vi "Insert Into Array (Boolean[]).vi"(9 "index":i32, 10 "Array":bool[](array[boolean]), 11 "JSON Value in":refnum<class "JSON Value.lvclass">) -> (3 "JSON Value out":refnum<class "JSON Value.lvclass">)   [LabVIEW 2017, in "JSON Value.lvclass"]
doc: "Inserts an element or subarray into a JSON array at the point you specify in index."
uses:
  JSON Value.lvclass
  Insert Into Array (Value[]).vi
  New JSON Value/New JSON (Boolean).vi
panel:
  out "error out":errorcluster
  in  "error in (no error)":errorcluster
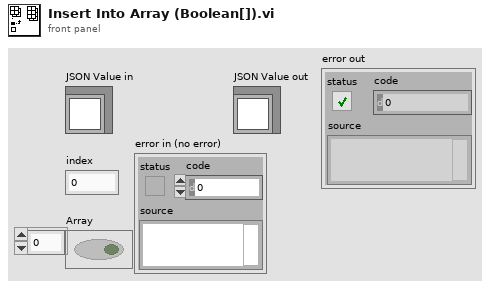
[diagram p1: front panel]
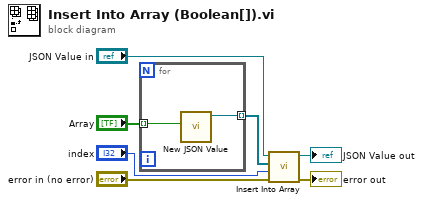
[diagram p0: block diagram]
diagram:
  n1 = for {
    tunnel: "Array" -> [w9] mode=indexing
    tunnel: [w8] -> w4 mode=indexing
    n2 = call-poly "New JSON Value.vi"("value"=w9) -> ("JSON Value out"=w8:refnum<class "JSON Value.lvclass">)  [unwired: 9 in, 1 out]
  }
  n3 = call-poly "Insert Into Array.vi"("error in (no error)"="error in (no error)", "index"="index", "Array"=w4, "JSON Array in"="JSON Value in") -> ("error out"=→"error out":errorcluster, "JSON Array out"=→"JSON Value out":refnum<class "JSON Value.lvclass">)  [unwired: 6 in]
